vi "RP_Eth.vi"() -> ()   [LabVIEW 2021]
panel:
  in  "port":u16
  in  "net address":u32
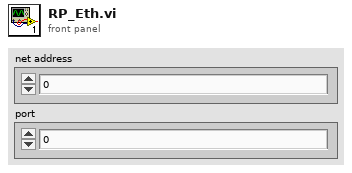
[diagram p1: front panel]
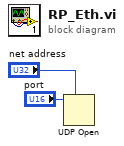
[diagram p0: block diagram]
diagram:
  n1 = UDP Open(7:"net address", 11:"port") -> ()  [unwired: 3 in, 3 out]
